vi "OAT Full Spectrum.vi"   [LabVIEW 2017, in "SoundVib_OrderTracking.lvlib"]
doc: "This VI computes the full spectrum of a probe pair. The full spectrum provides information on the amplitude of vibration as well as the orbit eccentricity and direction of precession for each frequency/order component."
uses:
  <vilib>/addons/Sound and Vibration/Order Analysis/Resample Order Tracking/SoundVib_OrderTracking.lvlib
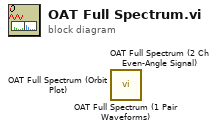
[diagram p0: block diagram]
diagram:
  n1 = call <vilib>:"OAT Full Spectrum (1 Pair Waveforms).vi"() -> ()  [unwired: 12 in, 8 out]
  n2 = call <vilib>:"OAT Full Spectrum (2 Ch Even-Angle Signal).vi"() -> ()  [unwired: 11 in, 9 out]
  n3 = call <vilib>:"OAT Full Spectrum (Orbit Plot).vi"() -> ()  [unwired: 14 in, 6 out]
